vi "Push.vi"(8 "error in (no error)":errorcluster, 10 "Element":dbl, 11 "UPNCalculator in":refnum<class "UPNCalculator.lvclass">) -> (0 "error out":errorcluster, 3 "UPNCalculator out":refnum<class "UPNCalculator.lvclass">)   [LabVIEW 2016, in "UPNCalculator Actor.lvlib" / "UPNCalculator.lvclass"]
doc: "Push an element on top of stack."
uses:
  UPNCalculator.lvclass
  UPNCalculator.lvclass/UPNCalculator.ctl
  Stack/Stack.lvclass
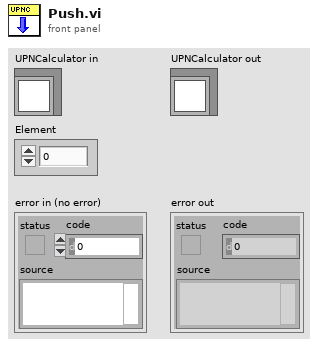
[diagram p1: front panel]
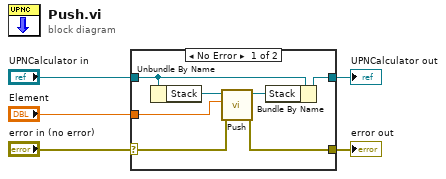
[diagram p0: block diagram]
diagram:
  n1 = case shown="No Error" "error in (no error)" {
    selector: "error in (no error)" -> [w10 w14]
    tunnel: [w9 w14] -> w4
    tunnel: [w6 w13] -> w2
    tunnel: "UPNCalculator in" -> [w7 w13]
    tunnel: "Element" -> [w11 _]
    frame No Error {
      n2 = Unbundle By Name(w7) -> ("Stack"=w12:refnum<class "Stack.lvclass">)
      n3 = call "Push.vi"("error in (no error)"=w10, "Element"=w11, "Stack in"=w12) -> ("error out"=w9:errorcluster, "Stack out"=w8:refnum<class "Stack.lvclass">)  [unwired: 7 in]
      n4 = Bundle By Name(cluster=w7, "Stack"=w8) -> (w6:refnum<class "UPNCalculator.lvclass">)
    }
    frame Error {
    }
  }
  "error out" <- w4
  "UPNCalculator out" <- w2
